vi "SeqGlobalVariable.vi"() -> ()   [LabVIEW 2017]
panel:
  in  "Seq":i32
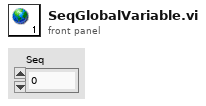
[diagram p1: front panel]
diagram:
